vi "CreateHeader.vi"(1 "Content":string) -> (0 "XML":string)   [LabVIEW 2015]
doc: "Creates an XML header"
uses:
  _ROSDefinition.vi
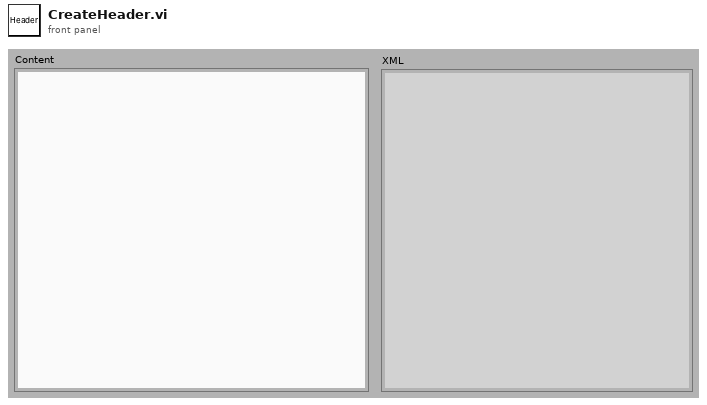
[diagram p1: front panel]
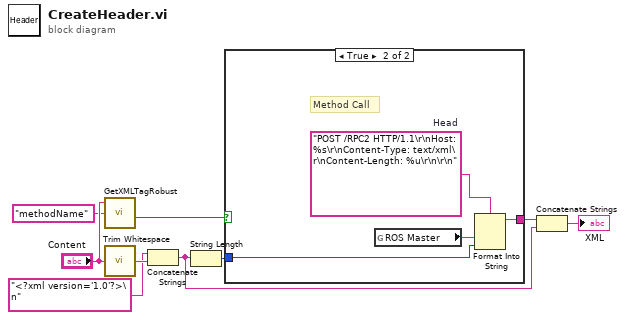
[diagram p0: block diagram]
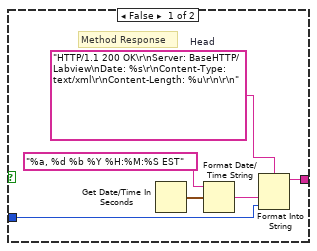
[diagram p2: hidden frame]
diagram:
  n1 = call "GetXMLTagRobust.vi"("Tag"="methodName", "String"="Content") -> ("Correct Tag Exists?"=w5:bool)  [unwired: 1 in, 3 out]
  n2 = call "Trim Whitespace.vi"("string"="Content") -> ("trimmed string"=w9:string)  [unwired: 1 in]
  n3 = Concatenate Strings("<?xml version='1.0'?>\n" ("string"), w9) -> (w2:string)
  n4 = String Length(string=w2) -> (length=w4:i32)
  n5 = case shown="True" w5 {
    tunnel: w4 -> [w11 w17]
    tunnel: [w10 w16] -> w3
    frame False {
      w15 = "HTTP/1.1 200 OK\r\nServer: BaseHTTP/Labview\nDate: %s\r\nContent-Type: text/xml\r\nContent-Length: %u\r\n\r\n"  # Head
      # "Method Response"
      n6 = Get Date/Time In Seconds() -> (seconds since 1Jan1904=w14:timestamp)
      n7 = Format Date/Time String(time format string (%c)="%a, %d %b %Y %H:%M:%S EST", seconds (now)=w14) -> (date/time string=w13:string)  [unwired: 1 in]
      n8 = Format Into String(format string=w15, w13, w11) -> (resulting string=w10:string)  [unwired: 2 in, 1 out]
    }
    frame True {
      w19 = "POST /RPC2 HTTP/1.1\r\nHost: %s\r\nContent-Type: text/xml\r\nContent-Length: %u\r\n\r\n"  # Head
      # "Method Call"
      n9 = global read "_ROSDefinition.vi" "ROS Master"() -> (w18:string)
      n10 = Format Into String(format string=w19, w18, w17) -> (resulting string=w16:string)  [unwired: 2 in, 1 out]
    }
  }
  n11 = Concatenate Strings(w3, w2) -> (→"XML":string)
